vi "remote.Get NVMEM Bytes.vi"(0 "SLSC Remote In":refnum<class "SLSC Remote.lvclass">, 5 "NVMEM area":refnum<k21>="$DefaultNVMEMAreas", 7 "data address":u32 format="%.0x", 9 "data size":u32, 11 "error in (no error)":errorcluster) -> (4 "SLSC Remote Out":refnum<class "SLSC Remote.lvclass">, 6 "NVMEM area out":refnum<k21>, 8 "next data address":u32 format="%.0x", 10 "data out":u8[](array[numeric]) format="%.0x", 15 "error out":errorcluster)   [LabVIEW 2016, in "SLSC Interfaces.lvlib" / "SLSC Remote.lvclass"]
uses:
  SLSC Remote.lvclass
  <vilib>/NI/NI JSONRPC Server Framework/Classes/Server/JSONRPC Server.lvclass
  <vilib>/httpClient/LabVIEWHTTPClient.lvlib
  <vilib>/httpClient/POSTBuffer.vi
  <vilib>/NI/JSON Support for LabVIEW/JSON Data Classes/JSON Helper/JSON Helper.lvclass
  <vilib>/NI/JSON Support for LabVIEW/JSON Data Classes/JSON Object/JSON Object.lvclass
  <vilib>/NI/JSON Support for LabVIEW/JSON Data Classes/JSON Helper/To More Specific Type (Object).vi
  <vilib>/NI/JSON Support for LabVIEW/JSON Data Classes/JSON Object/Get Value (Numeric Value).vi
  <vilib>/NI/JSON Support for LabVIEW/JSON Data Classes/JSON Object/New JSON Object (Empty).vi
  <vilib>/NI/JSON Support for LabVIEW/JSON Data Classes/JSON Object/Insert Key Value Pair (Single String).vi
  <vilib>/NI/JSON Support for LabVIEW/JSON Data Classes/JSON Object/Insert Key Value Pair (Single Numeric).vi
  <vilib>/NI/JSON Support for LabVIEW/JSON Data Classes/JSON Object/Get Value (String Value).vi
  <vilib>/NI/NI JSONRPC Server Framework/Classes/Server/Format Client Request (Auto-Increment).vi
  <vilib>/NI/NI JSONRPC Server Framework/Classes/Server/Parse Response (JSON).vi
  C:/Program Files (x86)/National Instruments/LabVIEW 2016/vi.lib/NI/JSON Support for LabVIEW/JSON Data Classes/JSON Structured Type/JSON Structure.lvclass
  C:/Program Files (x86)/National Instruments/LabVIEW 2016/vi.lib/NI/JSON Support for LabVIEW/JSON Data Classes/JSON Datatype/JSON Null.lvclass
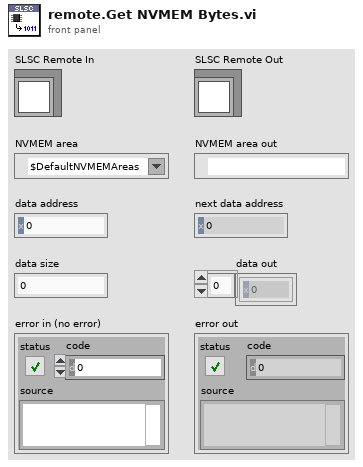
[diagram p1: front panel]
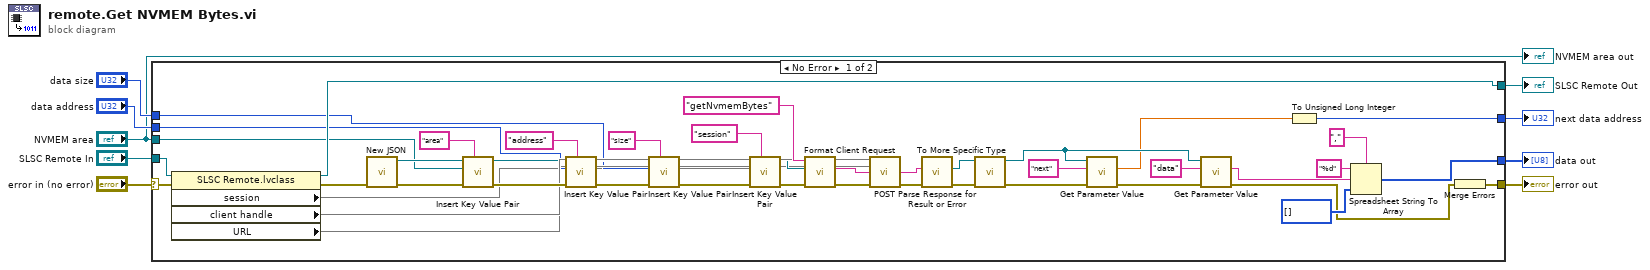
[diagram p0: block diagram]
diagram:
  n1 = case shown="No Error" "error in (no error)" {
    selector: "error in (no error)" -> [w53 w56]
    tunnel: "NVMEM area" -> [w20 _]
    tunnel: [w54 w55] -> w4
    tunnel: "data address" -> [w19 _]
    tunnel: "data size" -> [w18 _]
    tunnel: [w30 w56] -> w2
    tunnel: "SLSC Remote In" -> [w40 w55]
    tunnel: [w39 _] -> w3
    tunnel: [w13 _] -> w1
    frame No Error {
      n2 = property class="SLSC Remote.lvclass"(reference=w40, error in=w53) -> (reference out=w54:refnum<class "SLSC Remote.lvclass">, error out=w52:errorcluster, "session"=w17, "client handle"=w45, "URL"=w38)
      n3 = call-poly <vilib>:"New JSON.vi"("error in (no error)"=w52) -> ("error out"=w51:errorcluster, "JSON Object out"=w21:refnum<class "JSON Object.lvclass">)  [unwired: 9 in]
      n4 = call-poly <vilib>:"Insert Key Value Pair.vi"("key"="area" ("Name"), "error in (no error)"=w51, "value"=w20, "JSON Object in"=w21) -> ("error out"=w50:errorcluster, "JSON Object out"=w25:refnum<class "JSON Object.lvclass">)  [unwired: 5 in, 1 out]
      n5 = call-poly <vilib>:"Insert Key Value Pair.vi"("key"="address" ("Name"), "error in (no error)"=w50, "value"=w19, "JSON Object in"=w25) -> ("error out"=w47:errorcluster, "JSON Object out"=w24:refnum<class "JSON Object.lvclass">)  [unwired: 5 in, 1 out]
      n6 = call-poly <vilib>:"Insert Key Value Pair.vi"("key"="size" ("String"), "error in (no error)"=w47, "value"=w18, "JSON Object in"=w24) -> ("error out"=w46:errorcluster, "JSON Object out"=w23:refnum<class "JSON Object.lvclass">)  [unwired: 5 in, 1 out]
      n7 = call-poly <vilib>:"Insert Key Value Pair.vi"("key"="session" ("Name"), "error in (no error)"=w46, "value"=w17, "JSON Object in"=w23) -> ("error out"=w22:errorcluster, "JSON Object out"=w41:refnum<class "JSON Object.lvclass">)  [unwired: 5 in, 1 out]
      n8 = call-poly <vilib>:"Format Client Request.vi"("error in (no error)"=w22, "JSON in"=w41, "method"="getNvmemBytes") -> ("error out"=w44:errorcluster, "Request String"=w48:string)  [unwired: 7 in]
      n9 = call-poly <vilib>:"POST.vi"("client handle"=w45, "url"=w38, "buffer"=w48, "error in (no error)"=w44) -> ("body"=w43:string, "error out"=w42:errorcluster)  [unwired: 8 in, 2 out]
      n10 = call-poly <vilib>:"Parse Response for Result or Error.vi"("error in"=w42, "Response String In"=w43) -> ("error out"=w35:errorcluster, "JSON out"=w16:refnum<class "JSON Null.lvclass">)  [unwired: 7 in, 1 out]
      n11 = call-poly <vilib>:"To More Specific Type.vi"("error in (no error)"=w35, "JSON Datatype in"=w16) -> ("error out"=w36:errorcluster, "JSON Datatype out"=w33:refnum<class "JSON Object.lvclass">)  [unwired: 8 in]
      n12 = call-poly <vilib>:"Get Parameter Value.vi"("error in (no error)"=w36, "key"="next", "JSON Object in"=w33) -> ("error out"=w34:errorcluster, "value"=w31:dbl)  [unwired: 7 in]
      n13 = call-poly <vilib>:"Get Parameter Value.vi"("error in (no error)"=w34, "key"="data" ("Parameter Name"), "JSON Object in"=w33) -> ("error out"=w12:errorcluster, "value"=w15:string)  [unwired: 7 in]
      n14 = To Unsigned Long Integer(number=w31) -> (unsigned 32bit integer=w39:u32)
      n15 = Spreadsheet String To Array(delimiter (Tab)=",", format string="%d", spreadsheet string=w15, array type (2D Dbl)=u8[] [] ("data out")) -> (array=w13:u8[])
      n16 = Merge Errors(w12) -> (w30:errorcluster)
    }
    frame Error {
    }
  }
  "error out" <- w2
  "data out" <- w1
  "next data address" <- w3
  "SLSC Remote Out" <- w4
  "NVMEM area out" <- "NVMEM area"
